vi "Build_Row.vi"(8 "error in (no error)":errorcluster, 9 "Packet Number":i32, 11 "Ethernet frame":T1 {"fcs" format="%08x"; "network timestamp" format="%<%.7X\n%x>T"; "frame data" format="%x"; "local timestamp" format="%<%.7X\n%x>T"; "type" items=["Ethernet Data"=0, "Delay"=225, "Future Time Wait"=226]}) -> (0 "error out":errorcluster, 3 "Packet":string[](array[string]))   [LabVIEW 2025, in "Automotive Ethernet Bus Monitor.lvclass"]
uses:
  Automotive Ethernet Bus Monitor.lvclass
  <vilib>/xnet/xnet.llb/XNET Frame Ethernet.ctl
  <vilib>/xnet/xnet.llb/XNET Frame Type Ethernet.ctl
  Automotive Ethernet Bus Monitor.lvclass/Automotive Ethernet Bus Monitor.ctl
  Automotive Ethernet Bus Monitor UI/Automotive Ethernet Bus Monitor UI.lvlib
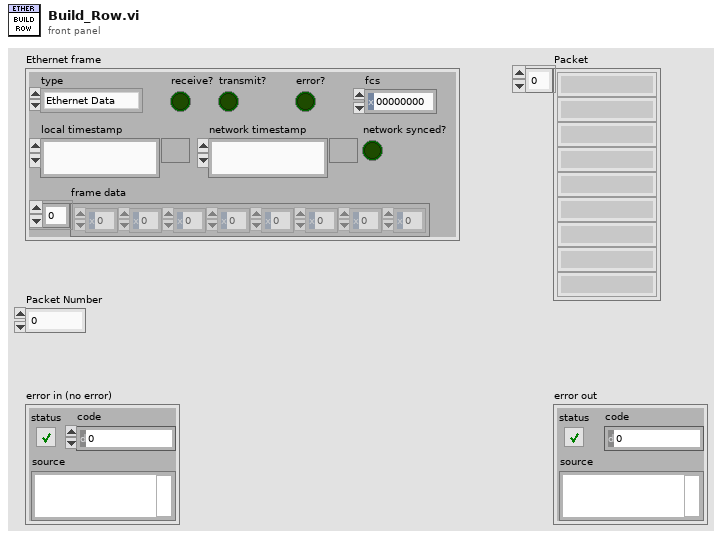
[diagram p1: front panel]
types:
  T1 = typedef "XNET Frame Ethernet.ctl" = cluster{"local timestamp":timestamp, "network timestamp":timestamp, "frame data":u8[], "fcs":u32, "type":T2, "network synced?":bool, "receive?":bool, "transmit?":bool, "error?":bool}
  T2 = typedef "XNET Frame Type Ethernet.ctl" = u16
  T3 = cluster{"destination MAC address":cluster{u8, u8, u8, u8, u8, u8}, "source MAC address":cluster{u8, u8, u8, u8, u8, u8}, "Has VLAN Tag":bool, "VLAN Tag":cluster{"TPID":u16, "priority":u8, "DEI":bool, "VID":u16}, "Ethertype":u16}
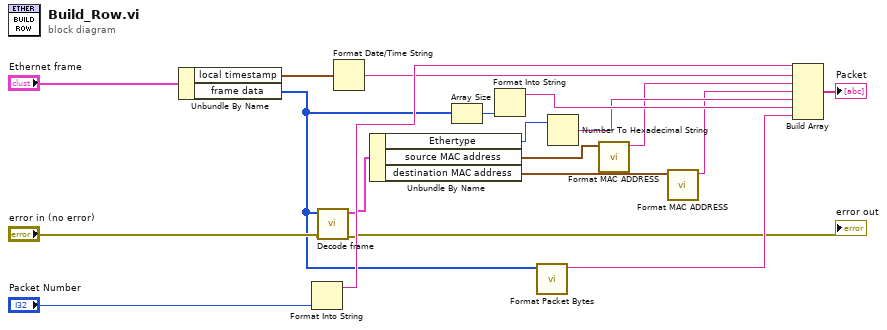
[diagram p0: block diagram]
diagram:
  n1 = Unbundle By Name("Ethernet frame") -> ("local timestamp"=w12:timestamp, "frame data"=w3:u8[])
  n2 = Format Into String("Packet Number") -> (resulting string=w19:string)  [unwired: 3 in, 1 out]
  n3 = call "Decode frame.vi"("error in (no error)"="error in (no error)", "frame data"=w3) -> ("error out"=→"error out":errorcluster, "Ethernet Header Cluster"=w2:T3)  [unwired: 7 in, 1 out]
  n4 = Format Date/Time String(seconds (now)=w12) -> (date/time string=w18:string)  [unwired: 2 in]
  n5 = Unbundle By Name(w2) -> ("Ethertype"=w14:u16, "source MAC address"=w9:cluster{u8, u8, u8, u8, u8, u8}, "destination MAC address"=w7:cluster{u8, u8, u8, u8, u8, u8})
  n6 = Array Size(array=w3) -> (size(s)=w17:i32)
  n7 = Format Into String(w17) -> (resulting string=w16:string)  [unwired: 3 in, 1 out]
  n8 = call "Format Packet Bytes.vi"("frame data"=w3) -> ("spreadsheet string"=w5:string)  [unwired: 10 in]
  n9 = Number To Hexadecimal String(2:w14) -> (0:w15:string)  [unwired: 1 in]
  n10 = call "Format MAC ADDRESS.vi"("source MAC address"=w9) -> ("spreadsheet string"=w8:string)  [unwired: 10 in]
  n11 = call "Format MAC ADDRESS.vi"("source MAC address"=w7) -> ("spreadsheet string"=w6:string)  [unwired: 10 in]
  n12 = Build Array(w19, w18, w8, w6, w15, w16, w5) -> (→"Packet":string[])
